vi "Set gain and speed.vi"(7 "EM on?":bool, 8 "error in (no error)":errorcluster, 9 "EM gain":i16, 10 "ADC gain":i16, 11 "camera handle in":i16) -> (0 "error out":errorcluster, 3 "camera handle out":i16)   [LabVIEW 2012]
uses:
  Visual Studio/Cascade wrapper/Release/Cascade wrapper.dll
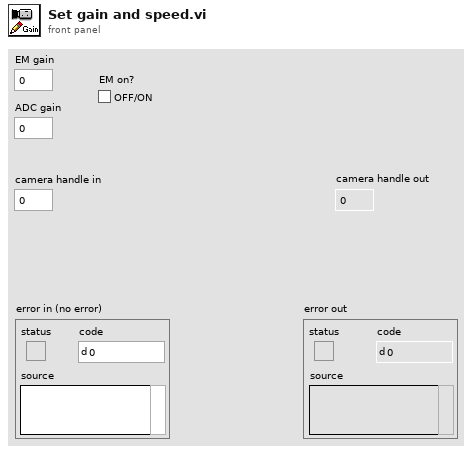
[diagram p1: front panel]
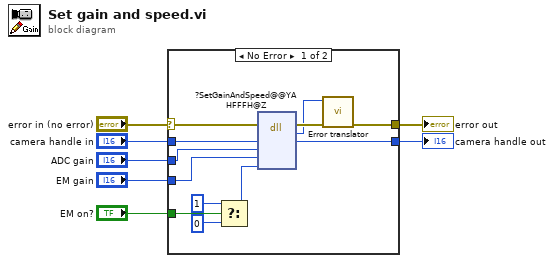
[diagram p0: block diagram]
diagram:
  n1 = case shown="No Error" "error in (no error)" {
    selector: "error in (no error)" -> [w15 w21]
    tunnel: "EM on?" -> [w19 _]
    tunnel: "camera handle in" -> [w14 w20]
    tunnel: "ADC gain" -> [w13 _]
    tunnel: "EM gain" -> [w12 _]
    tunnel: [w9 w21] -> w2
    tunnel: [w8 w20] -> w1
    frame No Error {
      n2 = Select(t=1, s=w19, f=0 ("t")) -> (s? t:f=w18:i32)
      n3 = dll-call lib="C:/moroder/Cascade wrapper/Visual Studio/Cascade wrapper/Release/Cascade wrapper.dll" fn="?SetGainAndSpeed@@YAHFFFH@Z"(error in=w15, "camera handle"=w14, "ADC gain"=w13, "EM gain"=w12, "EM on"=w18) -> (error out=w11:errorcluster, "error"=w10:i32, "camera handle"=w8:i16)  [unwired: 5 in, 1 out]
      n4 = call "Error translator.vi"("error in (no error)"=w11, "error code"=w10) -> ("error out"=w9:errorcluster)  [unwired: 9 in]
    }
    frame Error {
    }
  }
  "error out" <- w2
  "camera handle out" <- w1
